vi "Trigger Rolling Array (SubVI).vi"(0 "Waveform Input":waveform(dbl), 1 "Build Interval (ms)":u32, 2 "Max Elapsed Build Time (ms)":u32, 3 "Use Trigger SP?":bool, 4 "High Trigger SP (VDC)":dbl, 5 "Clear Trigger SP Latch":bool=TRUE) -> (16 "Waveform Array":T1(array[cluster]), 18 "Build Array Complete?":bool)   [LabVIEW 2009]
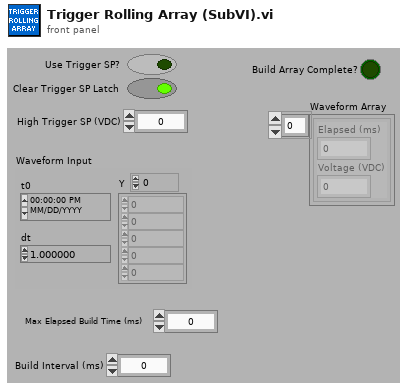
[diagram p1: front panel]
types:
  T1 = cluster{"Elapsed (ms)":u32, "Voltage (VDC)":dbl}[]
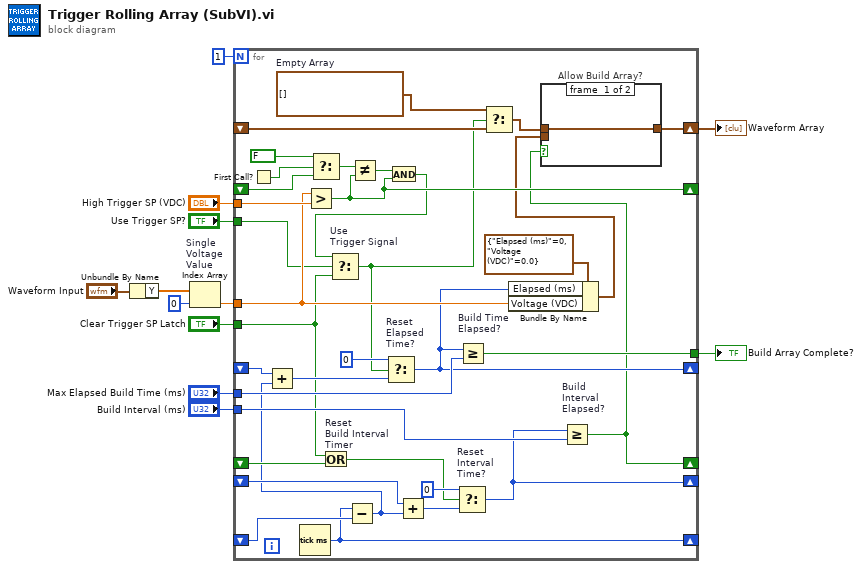
[diagram p0: block diagram]
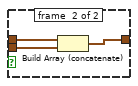
[diagram p2: hidden frame]
diagram:
  n1 = Unbundle By Name("Waveform Input") -> ("Y"=w7:dbl[])
  n2 = Index Array "Single\nVoltage\nValue"(array=w7, index=0) -> (element=w8:dbl)
  n3 = for {
    N: 1 -> [_]
    tunnel: "High Trigger SP (VDC)" -> [w46]
    shift-right: [w21] -> _
    shift-left: _ -> [w37]
    tunnel: w8 -> [w40]
    shift-right: [w38] -> w12
    shift-left: _ -> [w43]
    tunnel: "Max Elapsed Build Time (ms)" -> [w47]
    shift-right: [w23] -> _
    shift-left: _ -> [w42]
    shift-right: [w17] -> _
    shift-left: _ -> [w41]
    shift-right: [w13] -> _
    shift-left: _ -> [w32]
    tunnel: "Build Interval (ms)" -> [w24]
    tunnel: [w25] -> w3
    tunnel: "Clear Trigger SP Latch" -> [w18]
    shift-right: [w26] -> _
    shift-left: _ -> [w27]
    tunnel: "Use Trigger SP?" -> [w19]
    w16 = T1 []  # Empty Array
    n4 = First Call?() -> (First Call?: T/F=w35:bool)
    n5 = Tick Count (ms)() -> (millisecond timer value=w23:u32)
    n6 = Greater?(x=w40, y=w46) -> (0:w21:bool)
    n7 = Select(t=FALSE, s=w35, f=w37) -> (s? t:f=w36:bool)
    n8 = Or "Reset\nBuild Interval\nTimer"(x=w18, y=w32) -> (x .or. y?=w31:bool)
    n9 = Subtract(x=w23, y=w42) -> (x-y=w22:u32)
    n10 = Add(x=w27, y=w22) -> (x+y=w28:u32)
    n11 = Not Equal?(x=w36, y=w21) -> (x != y?=w45:bool)
    n12 = And(x=w45, y=w21) -> (x .and. y?=w20:bool)
    n13 = Select "Use\nTrigger Signal"(t=w20, s=w19, f=w18) -> (s? t:f=w15:bool)
    n14 = Select "Reset\nElapsed\nTime?"(t=u32 0, s=w15, f=w28) -> (s? t:f=w26:u32)
    n15 = Add(x=w41, y=w22) -> (x+y=w29:u32)
    n16 = Select "Reset\nInterval\nTime?"(t=u32 0, s=w31, f=w29) -> (s? t:f=w17:u32)
    n17 = Greater Or Equal? "Build Time\nElapsed?"(x=w26, y=w47) -> (x >= y?=w25:bool)
    n18 = Select(t=w16, s=w15, f=w43) -> (s? t:f=w39:T1)
    n19 = Bundle By Name(cluster=cluster{"Elapsed (ms)":u32, "Voltage (VDC)":dbl} {"Elapsed (ms)"=0, "Voltage (VDC)"=0.0}, "Elapsed (ms)"=w26, "Voltage (VDC)"=w40) -> (w14:cluster{"Elapsed (ms)":u32, "Voltage (VDC)":dbl})
    n20 = Greater Or Equal? "Build\nInterval\nElapsed?"(x=w17, y=w24) -> (x >= y?=w13:bool)
    n21 = case "Allow Build Array?" shown="True" w13 {
      tunnel: w14 -> [_ w49]
      tunnel: [w48 w51] -> w38
      tunnel: w39 -> [w48 w50]
      frame #0 {
      }
      frame #1 {
        n22 = Build Array (concatenate)(w50, w49) -> (w51:T1)
      }
    }
  }
  "Waveform Array" <- w12
  "Build Array Complete?" <- w3
